vi "Auto_Balance.vi"(1 "Timeout (ms)":dbl, 2 "Balance Complete Limit":dbl, 3 "Kp":dbl) -> ()   [LabVIEW 2020]
uses:
  <vilib>/Rock Robotics/WPI/ThirdParty/Phoenix-LabVIEW/Pigeon IMU/CTRE_PigeonIMU_GetYPR.vi
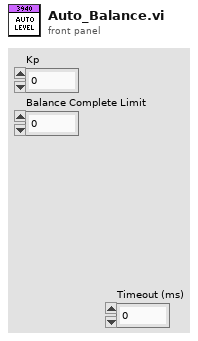
[diagram p1: front panel]
types:
  T1 = typedef "CTRE_PigeonIMU_DeviceRef.ctl" = cluster{"DeviceStatus":errorcluster, "Device Number":u8, "Type":T2, "Device ID":u32, "Handle":u64, "UsageFrame":u32, "Library Path":path}
  T2 = typedef "CTRE_PigeonIMU_ConnectionType.ctl" = u32
  T3 = typedef "WPI_RobotDriveDevRef.ctl" = cluster{"DevStatus":errorcluster, "Motors[]":T4[], "Square Inputs":bool, "Max Output":dbl}
  T4 = typedef "WPI_MotorControlDeviceRef.ctl" = cluster{"DeviceStatus":errorcluster, "Type":T5, "PWM":cluster{"PWM Channel":T6, "DeadBand":T7}, "CAN":cluster{"Device Number":u8, "SetOutput VI Ref":variant, "GetOutput VI Ref":variant, "Enable VI Ref":variant, "Disable VI Ref":variant, "Data":variant}, "Invert":bool, "DIO PWM":cluster{"PWM \"Enable\" Channel":T6, "DIOChannel":T8, "PWM Rate":dbl}}
  T5 = typedef "WPI_MotorControlType.ctl" = enum16{"PWM", "CAN", "DIO PWM"}
  T6 = typedef "FPGA_DIOPWMChannel.ctl" = enum8{"PWM 0", "PWM 1", "PWM 2", "PWM 3", "PWM 4", "PWM 5", "PWM 6", "PWM 7", "PWM 8", "PWM 9", "PWM MXP 0", "PWM MXP 1", "PWM MXP 2", "PWM MXP 3", "PWM MXP 4", "PWM MXP 5", "PWM MXP 6", "PWM MXP 7", "PWM MXP 8", "PWM MXP 9", "Invalid"}
  T7 = typedef "WPI_PWMDeadband.ctl" = cluster{"Name":string, "maxPositivePwm":i32, "minPositivePwm":i32, "centerPwm":i32, "maxNegativePwm":i32, "minNegativePwm":i32, "angularRange":u16}
  T8 = typedef "FPGA_DIOChannel.ctl" = enum8{"DIO 0", "DIO 1", "DIO 2", "DIO 3", "DIO 4", "DIO 5", "DIO 6", "DIO 7", "DIO 8", "DIO 9", "DIO MXP 0", "DIO MXP 1", "DIO MXP 2", "DIO MXP 3", "DIO MXP 4", "DIO MXP 5", "DIO MXP 6", "DIO MXP 7", "DIO MXP 8", "DIO MXP 9", "DIO MXP 10", "DIO MXP 11", "DIO MXP 12", "DIO MXP 13", "DIO MXP 14", "DIO MXP 15", "SPI Port CS1", "SPI Port CS2", "SPI Port CS3", "SPI Port MISO", "SPI Port MOSI", "Invalid"}
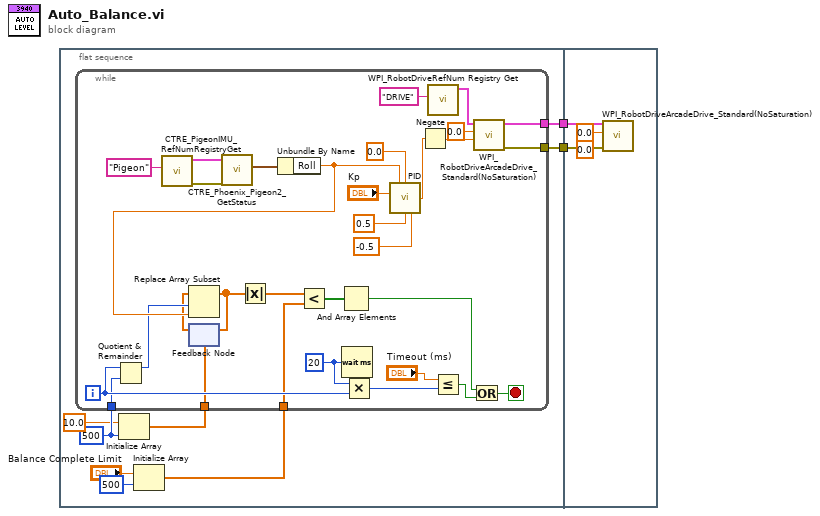
[diagram p0: block diagram]
diagram:
  n1 = flat-sequence {
    tunnel: [w4] -> w2
    tunnel: [w3] -> w1
    tunnel: w2 -> [w45]
    tunnel: w1 -> [w44]
    frame #0 {
      w10 = 500 ("dimension size")
      n2 = Initialize Array(10.0 ("element"), w10) -> (w8:dbl[])
      n3 = Initialize Array("Balance Complete Limit", 500 ("dimension size")) -> (w5:dbl[])
      n4 = while {
        tunnel: w10 -> [w22]
        tunnel: w8 -> [w18]
        tunnel: w5 -> [w15]
        tunnel: [w12] -> w4
        tunnel: [w11] -> w3
        i -> [w23]
        stop <- w37 stop-if-true
        w41 = u32 20 ("milliseconds to wait")
        n5 = Quotient & Remainder(x=w23, y=w22) -> (x-y*floor(x/y)=w20:i32)  [unwired: 1 out]
        n6 = call <vilib>:"CTRE_PigeonIMU_RefNumRegistryGet.vi"("refnum name"="Pigeon") -> ("error out"=w36:errorcluster, "PigeonIMUDevRef"=w35:T1)  [unwired: 9 in]
        n7 = feedback #1(w18) -> (w19:dbl[])
        n8 = call-poly <vilib>:"CTRE_Phoenix_Pigeon2_GetStatus.vi"("error in (no error)"=w36, "PigeonIMUDevRef"=w35) -> ("Yaw Pitch Roll"=w33:cluster{"Yaw":dbl, "Pitch":dbl, "Roll":dbl})  [unwired: 7 in, 2 out]
        n9 = Unbundle By Name(w33) -> ("Roll"=w21:dbl)
        n10 = Replace Array Subset(array=w19, new element=w21, index=w20) -> (w17:dbl[])
        n11 = feedback-in #1(w17) -> ()
        n12 = Absolute Value(x=w17) -> (abs(x)=w16:dbl[])
        n13 = Less?(x=w16, y=w15) -> (x < y?=w14:bool[])
        n14 = And Array Elements(Boolean array=w14) -> (logical AND=w13:bool)
        n15 = Wait (ms)(milliseconds to wait=w41) -> ()  [unwired: 1 out]
        n16 = Multiply(x=w41, y=w23) -> (x*y=w40:u32)
        n17 = call "PID.vi"("Kp"="Kp", "Process Variable"=w21, "Goal"=0.0, "Max Ouput"=0.5, "Min Output"=-0.5) -> ("Command"=w29:dbl)  [unwired: 8 in, 2 out]
        n18 = Negate(x=w29) -> (-x=w27:dbl)
        n19 = call <vilib>:"WPI_RobotDriveRefNum Registry Get.vi"("refnum name"="DRIVE") -> ("RobotDriveDevRef"=w25:T3)  [unwired: 9 in, 1 out]
        n20 = Less Or Equal?(x="Timeout (ms)", y=w40) -> (x <= y?=w38:bool)
        n21 = Or(x=w13, y=w38) -> (x .or. y?=w37:bool)
        n22 = call <vilib>:"WPI_RobotDriveArcadeDrive_Standard(NoSaturation).vi"("Y axis value"=w27, "X axis value"=0.0, "RobotDriveDevRef"=w25) -> ("error out"=w11:errorcluster, "RobotDriveDevRef"=w12:T3)  [unwired: 1 in, 6 out]
      }
    }
    frame #1 {
      n23 = call <vilib>:"WPI_RobotDriveArcadeDrive_Standard(NoSaturation).vi"("error in (no error)"=w44, "Y axis value"=0.0, "X axis value"=0.0, "RobotDriveDevRef"=w45) -> ()  [unwired: 8 out]
    }
  }
